vi "Vision Research Phantom Series PhCon PhCineSet.vi"(0 "CN [in]":u32, 1 "Cine":i32, 2 "Sel":T1 items=["cgsVideoTone"=4097, "cgsName"=4098, "cgsVideoMarkIn"=4099, "cgsVideoMarkOut"=4100, "cgsIsRecorded"=4101, "cgsHqMode"=4102, "cgsBurstCount"=4103, "cgsBurstPeriod"=4104, "cgsLensDescription"=4105, "cgsLensAperature"=4106, "cgsLensFocalLength"=4107, "cgsShutterOff"=4108, "cgsTriggerTime"=4109, "cgsTrigTC"=4110, "cgsPbRate"=4111, "cgsTcRate"=4112, "cgsWb"=5100, "cgsBright"=5101, "cgsContrast"=5102, "cgsGamma"=5103, "cgsGammaR"=5109, "cgsGammaB"=5110, "cgsSaturation"=5104, "cgsHue"=5105, "cgsPedestalR"=5106, "cgsPedestalG"=5107, "cgsPedestalB"=5108, "cgsFlare"=5111, "cgsChroma"=5112, "cgsTone"=5113, "cgsUserMatrix"=5114, "cgsEnableMatrices"=5115], 3 "pVal [in]":u64, 5 "Error In (no error)":errorcluster) -> (14 "CN [out]":u32=1, 15 "pVal [out]":u64, 19 "Error Out":errorcluster)   [LabVIEW 2013, in "VRI.lvlib"]
doc: "PhCineSet\nHRESULT PhCineSet(UNIT CN, INT Cine, UINT Sel, PVOID pVal);\n\nParameters\nCN [in]\n Camera number.\nCine [in]\n Cine number.\nSel [in]\n Numerical selector identifying the parameter to be set.\npVal [in, out]\n Input: value to be set.\n Output: accepted value for the cine parameter.\n\nReturn Value\nThe function returns ERR_Ok in case of success or an error code, otherwise. To get extended error information call PhGetErrorMessage.\n\nRemarks\nSets requested information for the specified camera cine. The cine is identified based on a cine number and the camera number it belongs to.\nPlease note that the last parameter must be passed by reference. The function will return back to the caller accepted value for the specified cine parameter.\nCheck Appendix 3 for possible selector values.\nImportant! This is a low level function. Use it only if neither PhSetCineInfo nor PhSetCineParams/PhSetSingleCineParams can provide needed functionality. There is no interaction between this function and CINEHANDLE objects!\n\nRequired Header\nPhCon.h"
uses:
  VRI.lvlib
  _Type Defs/PhCon CGS.ctl
  Phantom DLLs/PhCon.dll
panel:
  # "For instructions on the use of this VI, press Ctrl+H to display the help window and move the mouse over the icon, controls, and indicators"
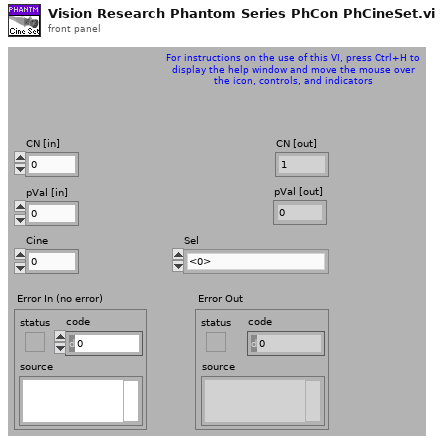
[diagram p1: front panel]
types:
  T1 = typedef "VRI.lvlib/PhCon CGS.ctl" = u16
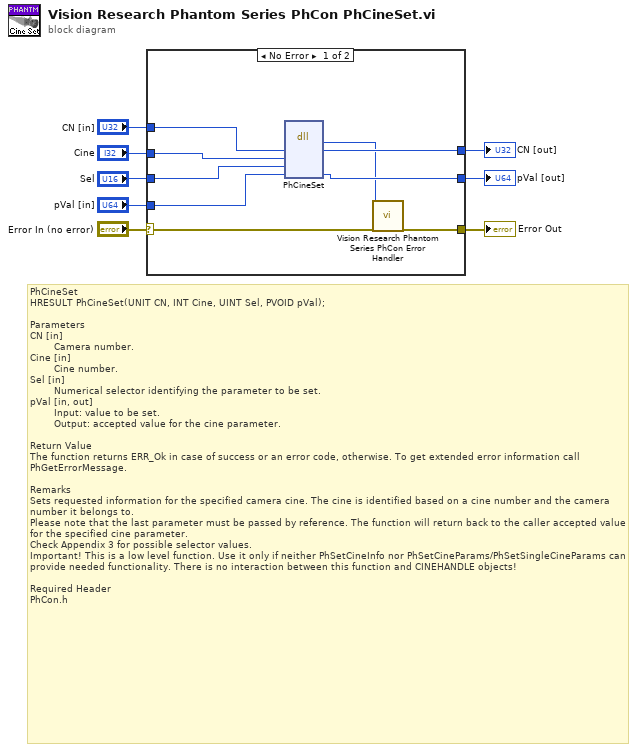
[diagram p0: block diagram]
diagram:
  # "PhCineSet\nHRESULT PhCineSet(UNIT CN, INT Cine, UINT Sel, PVOID pVal);\n\nParameters\nCN [in]\n\t       Camera number.\nCine [in]\n\t\t      Cine number.\nSel [in]\n\t\t      Numerical selector identifying the parameter to be set.\npVal [in, out]\n\t\t      Input: value to be set.\n\t\t      Output: accepted value for the cine parameter.\n\nReturn Value\nThe function returns ERR_Ok in case of success or an error code, otherwise. To get extended error information call PhGetErrorMessage.\n\nRemarks\nSets requested information for the specified camera cine. The cine is identified based on a cine number and the camera number it belongs to.\nPlease note that the last parameter must be passed by reference. The function will return back to the caller accepted value for the specified cine parameter.\nCheck Appendix 3 for possible selector values.\nImportant! This is a low level function. Use it only if neither PhSetCineInfo nor PhSetCineParams/PhSetSingleCineParams can provide needed functionality. There is no interaction between this function and CINEHANDLE objects!\n\nRequired Header\nPhCon.h"
  n1 = case shown="No Error" "Error In (no error)" {
    selector: "Error In (no error)" -> [w17 w20]
    tunnel: [w16 w20] -> w7
    tunnel: "CN [in]" -> [w15 w19]
    tunnel: [w14 w19] -> w5
    tunnel: "Sel" -> [w13 _]
    tunnel: "Cine" -> [w12 _]
    tunnel: "pVal [in]" -> [w11 w18]
    tunnel: [w10 w18] -> w1
    frame No Error {
      n2 = dll-call lib="C:/Projects/SDK/32-bit/Vision Research Phantom Series Labview Driver/Phantom DLLs/PhCon.dll" fn="PhCineSet"("CN"=w15, "Cine"=w12, "Sel"=w13, "pVal"=w11) -> ("HRESULT"=w9:i32, "CN"=w14:u32, "pVal"=w10:u64)  [unwired: 4 in, 3 out]
      n3 = call "Vision Research Phantom Series PhCon Error Handler.vi"("ErrNo"=w9, "Error In (no error)"=w17) -> ("Error Out"=w16:errorcluster)  [unwired: 17 out]
    }
    frame Error {
    }
  }
  "Error Out" <- w7
  "CN [out]" <- w5
  "pVal [out]" <- w1
